vi "Stop Core.vi"(10 "final error code":i32, 11 "TCPIP Communications in":refnum<class "TCPIP Communications.lvclass">) -> (3 "TCPIP Communications out":refnum<class "TCPIP Communications.lvclass">)   [LabVIEW 2015, in "TCPIP Communications Framework.lvlib" / "TCPIP Communications.lvclass"]
doc: "(<B>Filename</B>: Actor Framework.lvlib:Actor.lvclass:Stop Core.vi)\n\nDefines what the actor does before it stops. Use the <B>final error code</B> input to determine whether the actor shut down in response to an error.\n\nBy default, this method does nothing. A descendant class may override it to define behavior, such as shutting down any processes the actor initiated in its override of the Actor Core method."
uses:
  TCPIP Communications.lvclass
  <vilib>/ActorFramework/Actor/Actor.lvclass
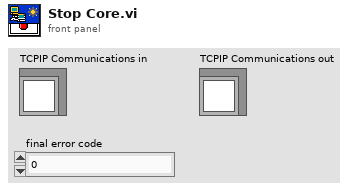
[diagram p1: front panel]
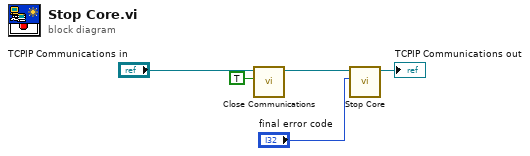
[diagram p0: block diagram]
diagram:
  n1 = call-dynamic "Close Communications.vi"("Final Stop?"=TRUE, "TCPIP Communications in"="TCPIP Communications in") -> ("TCPIP Communications out"=w2:refnum<class "TCPIP Communications.lvclass">)  [unwired: 8 in, 1 out]
  n2 = call-parent "Stop Core.vi"("final error code"="final error code", "Actor in"=w2) -> ("Actor out"=→"TCPIP Communications out":refnum<class "TCPIP Communications.lvclass">)  [unwired: 9 in]
